vi "HeightShooter.vi"() -> ()   [LabVIEW 2013]
panel:
  out "shooter height":dbl
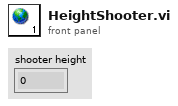
[diagram p1: front panel]
diagram:
